vi "Motion設定轉換.vi"(5 "速度模式":bool, 7 "速度分段":enum16{"低速", "中速", "高速"}(ring), 8 "速度 in":i32, 9 "旋轉移動角度":i32, 10 "位置移動距離":i32, 11 "Axis Ring in":i32) -> (1 "速度 out":i32=1000 min=0 max=3000, 2 "移動":i32(ring) items=["0.01 mm", "0.1 mm", "1 mm", "10 mm"], 3 "Axis Ring out":i32(ring) items=["01A-1 Å|Tray¤J®Æ(Step)", "01A-2 空Tray疊盤(Step)", "02A-1 取料移載-X(Step)", "02A-2取料移載-Y(Step)", "02A-3 CCD對位移載-X(Step01)", "02A-4 CCD對位移載-X(Step02)", "02A-5 CCD對位移載-Y(Servo)", "02A-6 對位-θ(Step01)", "02A-7 對位-θ(Step02)", "04A-1 Glue-對位-X(Step)", "04A-2 Glue-對位-Y(Step)", "05A-1 UV-對位-X(Step)", "05A-2 UV-對位-Y(Step)", "08A-1 噴頭移載(Step)", "09A-1 移載退料-X(Step)", "09A-2 移載退料-Y(Servo)", "09A-3 調夾距(Step)", "09A-4 退料R(Step)", "10A-1 空Tray入料(Step)", "10A-2 滿Tray出料(Step)", ""])   [LabVIEW 2015]
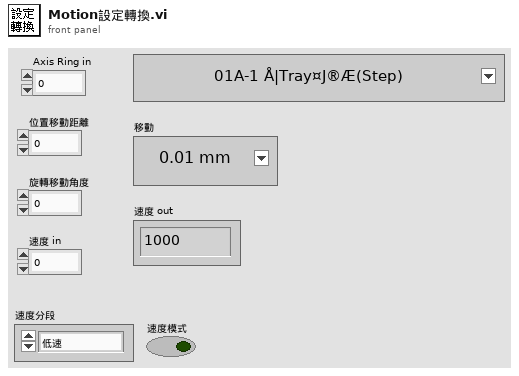
[diagram p1: front panel]
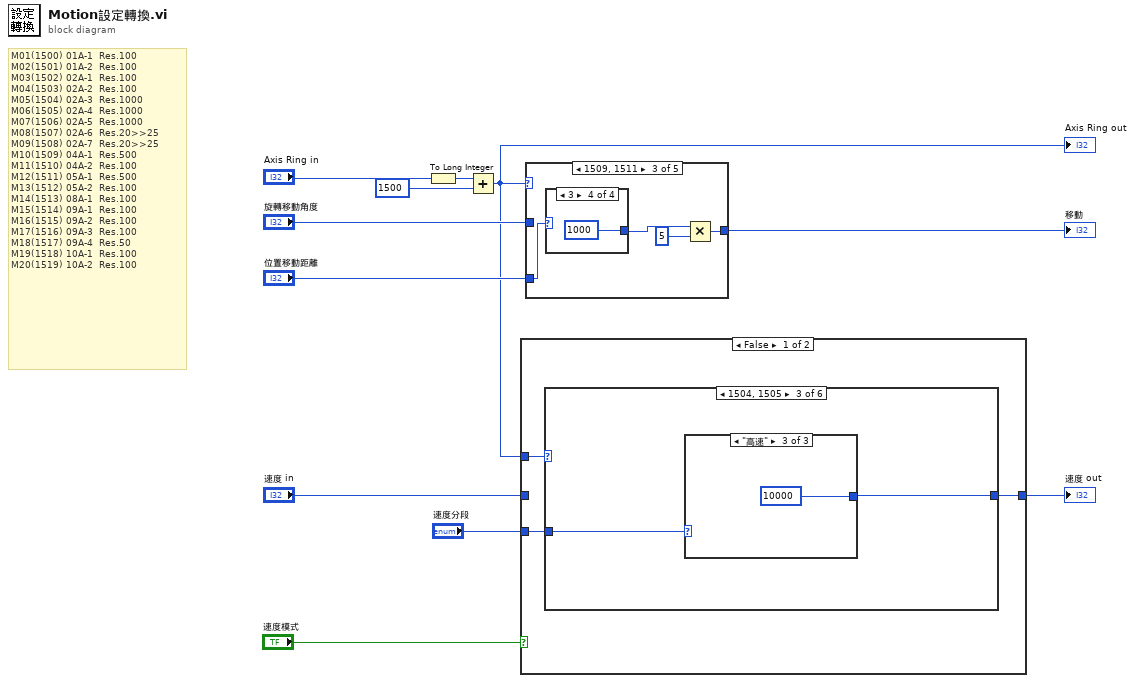
[diagram p0: block diagram]
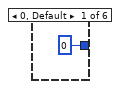
[diagram p2: hidden frame]
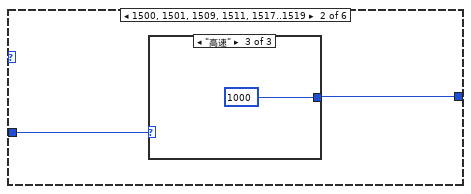
[diagram p3: hidden frame]
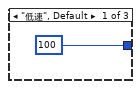
[diagram p4: hidden frame]
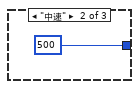
[diagram p5: hidden frame]
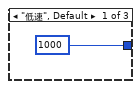
[diagram p6: hidden frame]
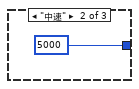
[diagram p7: hidden frame]
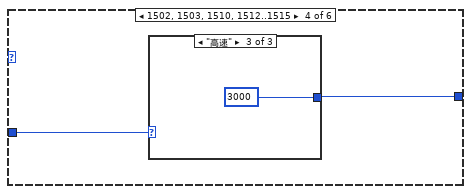
[diagram p8: hidden frame]
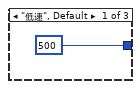
[diagram p9: hidden frame]
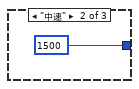
[diagram p10: hidden frame]
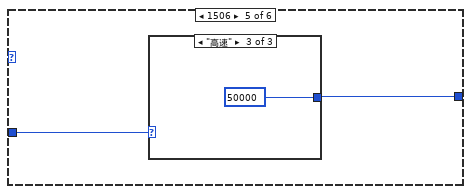
[diagram p11: hidden frame]
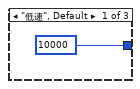
[diagram p12: hidden frame]
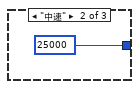
[diagram p13: hidden frame]
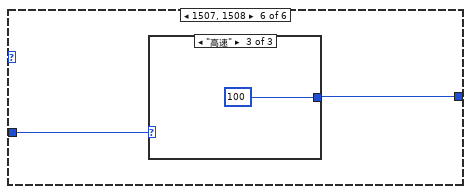
[diagram p14: hidden frame]
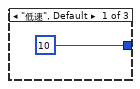
[diagram p15: hidden frame]
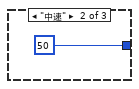
[diagram p16: hidden frame]
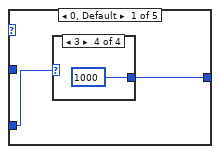
[diagram p18: hidden frame]
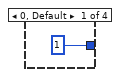
[diagram p19: hidden frame]
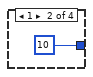
[diagram p20: hidden frame]
diagram:
  # "M01(1500) 01A-1  Res.100\nM02(1501) 01A-2  Res.100\nM03(1502) 02A-1  Res.100\nM04(1503) 02A-2  Res.100\nM05(1504) 02A-3  Res.1000\nM06(1505) 02A-4  Res.1000\nM07(1506) 02A-5  Res.1000\nM08(1507) 02A-6  Res.20>>25\nM09(1508) 02A-7  Res.20>>25\nM10(1509) 04A-1  Res.500\nM11(1510) 04A-2  Res.100\nM12(1511) 05A-1  Res.500\nM13(1512) 05A-2  Res.100\nM14(1513) 08A-1  Res.100\nM15(1514) 09A-1  Res.100\nM16(1515) 09A-2  Res.100\nM17(1516) 09A-3  Res.100\nM18(1517) 09A-4  Res.50\nM19(1518) 10A-1  Res.100\nM20(1519) 10A-2  Res.100"
  n1 = To Long Integer(number="Axis Ring in") -> (32bit integer=w9:i32)
  n2 = Add(x=w9, y=1500) -> (x+y=w2:i32)
  "Axis Ring out" <- w2
  n3 = case shown="False" "速度模式" {
    tunnel: [w13 w41] -> w4
    tunnel: "速度 in" -> [_ w41]
    tunnel: w2 -> [w14 _]
    tunnel: "速度分段" -> [w12 _]
    frame False {
      n4 = case shown="1504, 1505" w14 {
        tunnel: [0 w17 w22 w27 w32 w37] -> w13
        tunnel: w12 -> [_ w16 w21 w26 w31 w36]
        frame 0, Default {
        }
        frame 1500, 1501, 1509, 1511, 1517..1519 {
          n5 = case shown="\"高速\"" w16 {
            tunnel: [100 500 1000] -> w17
            frame "低速", Default {
            }
            frame "中速" {
            }
            frame "高速" {
            }
          }
        }
        frame 1504, 1505 {
          n6 = case shown="\"高速\"" w21 {
            tunnel: [1000 5000 10000] -> w22
            frame "低速", Default {
            }
            frame "中速" {
            }
            frame "高速" {
            }
          }
        }
        frame 1502, 1503, 1510, 1512..1515 {
          n7 = case shown="\"高速\"" w26 {
            tunnel: [500 1500 3000] -> w27
            frame "低速", Default {
            }
            frame "中速" {
            }
            frame "高速" {
            }
          }
        }
        frame 1506 {
          n8 = case shown="\"高速\"" w31 {
            tunnel: [10000 25000 50000] -> w32
            frame "低速", Default {
            }
            frame "中速" {
            }
            frame "高速" {
            }
          }
        }
        frame 1507, 1508 {
          n9 = case shown="\"高速\"" w36 {
            tunnel: [10 50 100] -> w37
            frame "低速", Default {
            }
            frame "中速" {
            }
            frame "高速" {
            }
          }
        }
      }
    }
    frame True {
    }
  }
  "速度 out" <- w4
  n10 = case shown="1509, 1511" w2 {
    tunnel: [w42 w48 w56 w65 w71] -> w8
    tunnel: "旋轉移動角度" -> [_ _ _ w64 w72]
    tunnel: "位置移動距離" -> [w43 w51 w59 _ _]
    frame 0, Default {
      n11 = case shown="3" w43 {
        tunnel: [1 ("y") 10 ("y") 100 ("y") 1000 ("y")] -> w42
        frame 0, Default {
        }
        frame 1 {
        }
        frame 2 {
        }
        frame 3 {
        }
      }
    }
    frame 1506 {
      n12 = case shown="3" w51 {
        tunnel: [1 ("y") 10 ("y") 100 ("y") 1000 ("y")] -> w50
        frame 0, Default {
        }
        frame 1 {
        }
        frame 2 {
        }
        frame 3 {
        }
      }
      n13 = Multiply(x=w50, y=10) -> (x*y=w48:i32)
    }
    frame 1509, 1511 {
      n14 = case shown="3" w59 {
        tunnel: [1 ("y") 10 ("y") 100 ("y") 1000 ("y")] -> w57
        frame 0, Default {
        }
        frame 1 {
        }
        frame 2 {
        }
        frame 3 {
        }
      }
      n15 = Multiply(x=w57, y=5) -> (x*y=w56:i32)
    }
    frame 1507, 1508 {
      n16 = case shown="0, Default" w64 {
        tunnel: [1 ("y") 10 ("y") 20 ("y") 200 ("y")] -> w65
        frame 0, Default {
        }
        frame 1 {
        }
        frame 2 {
        }
        frame 3 {
        }
      }
    }
    frame 1517 {
      n17 = case shown="1" w72 {
        tunnel: [1 ("y") 10 ("y") 100 ("y") 3600 ("y")] -> w73
        frame 0, Default {
        }
        frame 1 {
        }
        frame 2 {
        }
        frame 3 {
        }
      }
      n18 = Multiply(x=w73, y=5) -> (x*y=w71:i32)
    }
  }
  "移動" <- w8
